vi "Read Log File.vi"(8 "error in (no error)":errorcluster, 11 "Mag Lab Error Handler in":refnum<class "Mag Lab Error Handler.lvclass">) -> (0 "error out":errorcluster, 2 "Log File":path, 3 "Mag Lab Error Handler out":refnum<class "Mag Lab Error Handler.lvclass">)   [LabVIEW 2015, in "Mag Lab Error Handler.lvlib" / "Mag Lab Error Handler.lvclass"]
uses:
  Mag Lab Error Handler.lvclass
  Mag Lab Error Handler.lvclass/Mag Lab Error Handler.ctl
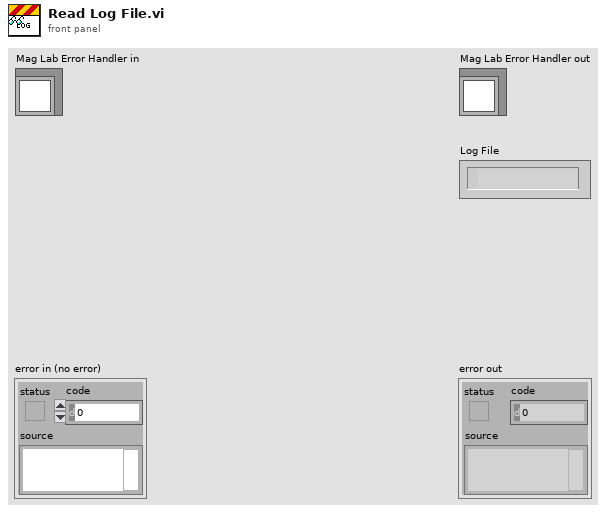
[diagram p1: front panel]
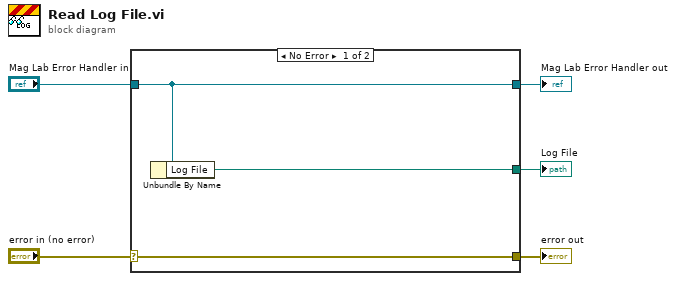
[diagram p0: block diagram]
diagram:
  n1 = case shown="No Error" "error in (no error)" {
    selector: "error in (no error)" -> [w8 w9]
    tunnel: [w8 w9] -> w4
    tunnel: [w7 w10] -> w2
    tunnel: "Mag Lab Error Handler in" -> [w7 w10]
    tunnel: [w6 _] -> w1
    frame No Error {
      n2 = Unbundle By Name(w7) -> ("Log File"=w6:path)
    }
    frame Error {
    }
  }
  "error out" <- w4
  "Mag Lab Error Handler out" <- w2
  "Log File" <- w1
